vi "espectroCCD.vi"(7 "Enable Strobe (Disabled)":bool, 8 "tiempo de lectura (ms)":u32, 9 "Numero de lecturas":i32, 11 "VISA resource name":refnum<visa-resource-name>) -> (1 "arreglo promedio":dbl[](array[numeric]), 3 "Wavelength (nm)":dbl[](array[numeric]))   [LabVIEW 2016]
doc: "En este subVI se obtienen los datos desde el espectrómetro CCD para que los muestre en una gráfica.\n\nSus entradas son los tiempos de lectura y el numero de lecturas a realizar, el VISA resource name y el habilitado del Strobe.\nSus salidas son un arreglo con las longitudes de onda y otro con las intensidades obtenidas."
uses:
  <vilib>/Analysis/baseanly.llb/Mean (DBL).vi
  <instrlib>/Ocean Optics 2000 4000/Ocean Optics 2000 4000.lvlib
  <vilib>/Analysis/NI_AALBase.lvlib
panel:
  out "Spectrum by Pixel Number":dbl[](array[numeric])
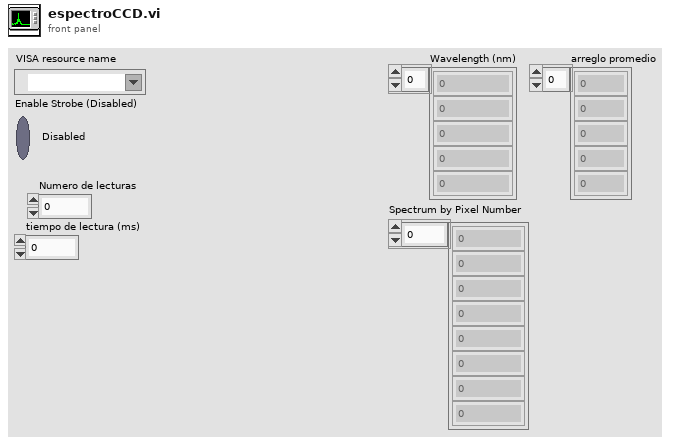
[diagram p1: front panel]
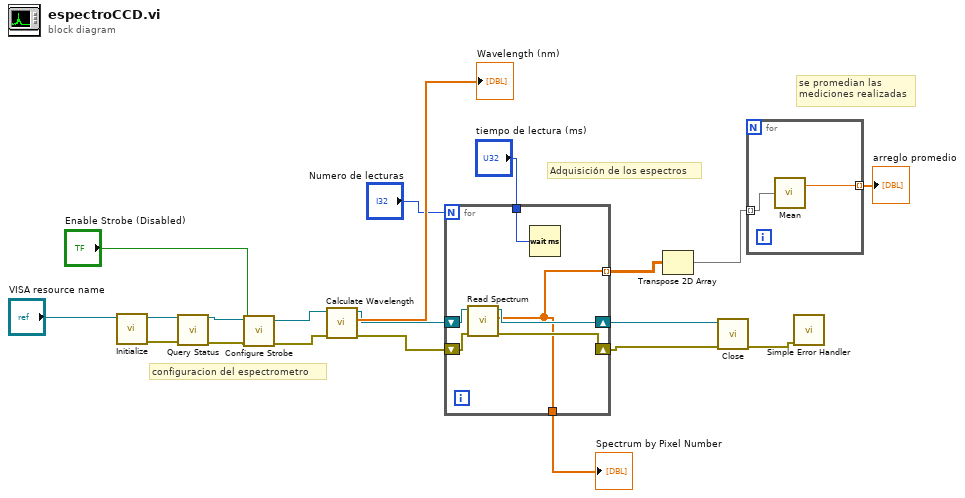
[diagram p0: block diagram]
diagram:
  # "configuracion del espectrometro"
  # "Adquisición de los espectros"
  # "se promedian las\nmediciones realizadas"
  n1 = call <instrlib>:"Initialize.vi"("VISA resource name"="VISA resource name") -> ("error out"=w18:errorcluster, "VISA resource name out"=w19:refnum<visa-resource-name>)  [unwired: 9 in]
  n2 = call <instrlib>:"Query Status.vi"("VISA resource name"=w19, "error in (no error)"=w18) -> ("VISA resource name out"=w17:refnum<visa-resource-name>, "error out"=w16:errorcluster)  [unwired: 6 in, 6 out]
  n3 = call <instrlib>:"Configure Strobe.vi"("error in (no error)"=w16, "Enable Strobe (Disabled)"="Enable Strobe (Disabled)", "VISA resource name"=w17) -> ("error out"=w13:errorcluster, "VISA resource name out"=w14:refnum<visa-resource-name>)  [unwired: 7 in]
  n4 = call <instrlib>:"Calculate Wavelength.vi"("error in (no error)"=w13, "VISA resource name"=w14) -> ("error out"=w10:errorcluster, "Wavelength (nm)"=→"Wavelength (nm)":dbl[], "VISA resource name out"=w11:refnum<visa-resource-name>)  [unwired: 7 in]
  n5 = for {
    N: "Numero de lecturas" -> [_]
    tunnel: [w21] -> w7
    shift-right: [w24] -> w9
    shift-left: w11 -> [w26]
    shift-right: [w23] -> w8
    shift-left: w10 -> [w25]
    tunnel: "tiempo de lectura (ms)" -> [w22]
    tunnel: [w21] -> w3 mode=indexing
    n6 = call <instrlib>:"Read Spectrum.vi"("error in (no error)"=w25, "VISA resource name"=w26) -> ("error out"=w23:errorcluster, "Spectrum by Pixel Number"=w21:dbl[], "VISA resource name out"=w24:refnum<visa-resource-name>)  [unwired: 6 in, 1 out]
    n7 = Wait (ms)(milliseconds to wait=w22) -> ()  [unwired: 1 out]
  }
  "Spectrum by Pixel Number" <- w7
  n8 = Transpose 2D Array(2D array=w3) -> (transposed array=w2:dbl[][])
  n9 = call <instrlib>:"Close.vi"("error in (no error)"=w8, "VISA resource name"=w9) -> ("error out"=w1:errorcluster)  [unwired: 9 in]
  n10 = for {
    tunnel: w2 -> [w28] mode=indexing
    tunnel: [w27] -> w4 mode=indexing
    n11 = call-poly <vilib>:"Mean.vi"("X"=w28) -> ("mean"=w27:dbl)  [unwired: 1 out]
  }
  "arreglo promedio" <- w4
  n12 = call <vilib>:"Simple Error Handler.vi"("error in (no error)"=w1) -> ()  [unwired: 4 in, 5 out]
